vi "Read Transport.vi"(11 "Attributes in":refnum<class "Attributes.lvclass">) -> (2 "Transport":refnum<class "Transport.lvclass">)   [LabVIEW 2020, in "jettl.lvlib" / "Attributes.lvclass"]
uses:
  Attributes.lvclass
  Transport/Transport.lvclass
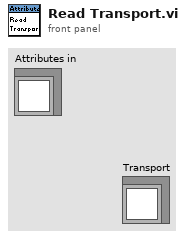
[diagram p1: front panel]
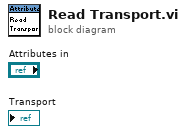
[diagram p0: block diagram]
diagram:
